vi "DataFolder.vi"() -> (2 "appended path":path)   [LabVIEW 2016]
uses:
  <vilib>/Utility/sysdir.llb/System Directory Type.ctl
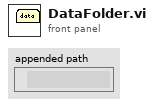
[diagram p1: front panel]
types:
  T1 = enum32{"invalid app kind", "Development System", "Run Time System", "Student Edition", "Embedded LabVIEW", "Evaluation", "Custom"}
  T2 = typedef "System Directory Type.ctl" = i32
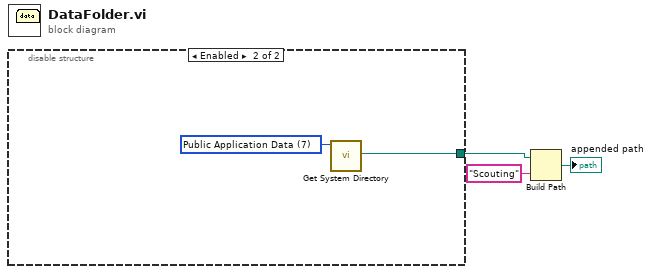
[diagram p0: block diagram]
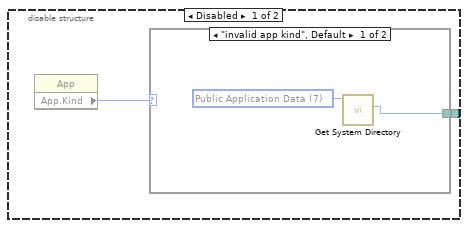
[diagram p2: hidden frame]
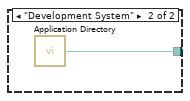
[diagram p3: hidden frame]
diagram:
  n1 = disable-structure shown="Enabled" {
    disable-tunnel: [w4 w9] -> w3
    frame Disabled {
      n2 = property class="App"() -> ("App.Kind"=w5:T1)  [unwired: 2 in, 2 out]
      n3 = case shown="\"invalid app kind\", Default" w5 {
        tunnel: [w6 w8] -> w4
        frame "invalid app kind", Default {
          w7 = T2 7 items=["User Home"=0, "User Desktop"=1, "User Documents"=2, "User Application Data"=3, "User Preferences"=4, "User Temporary"=5, "Public Documents"=6, "Public Application Data"=7, "Public Preferences"=8, "Public Cache"=13, "System Core Libraries"=9, "System Installed Libraries"=10, "Application Files"=11, "Boot Volume Root"=12] ("system directory type")
          n4 = call <vilib>:"Get System Directory.vi"("system directory type"=w7) -> ("system directory"=w6:path)  [unwired: 10 in]
        }
        frame "Development System" {
          n5 = call <vilib>:"Application Directory.vi"() -> ("Application Directory"=w8:path)
        }
      }
    }
    frame Enabled {
      w10 = T2 7 items=["User Home"=0, "User Desktop"=1, "User Documents"=2, "User Application Data"=3, "User Preferences"=4, "User Temporary"=5, "Public Documents"=6, "Public Application Data"=7, "Public Preferences"=8, "Public Cache"=13, "System Core Libraries"=9, "System Installed Libraries"=10, "Application Files"=11, "Boot Volume Root"=12] ("system directory type")
      n6 = call <vilib>:"Get System Directory.vi"("system directory type"=w10) -> ("system directory"=w9:path)  [unwired: 10 in]
    }
  }
  n7 = Build Path(base path=w3, name or relative path="Scouting") -> (appended path=→"appended path":path)
